vi "libzmq path.vi"() -> (2 "path":path)   [LabVIEW 2019, in "RemoteControl.ZMQ.lvlib" / "RemoteControl.ZMQ.lvclass"]
uses:
  RemoteControl.ZMQ.lvclass
  libzmq/libzmq.lvclass
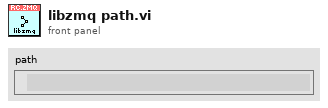
[diagram p1: front panel]
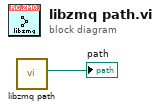
[diagram p0: block diagram]
diagram:
  n1 = call "libzmq path.vi"() -> ("path"=→"path":path)  [unwired: 11 in]
